vi "TEST - Copy with Options.vi"(8 "error in (no error)":errorcluster) -> (0 "error out":errorcluster, 2 "pass":bool)   [LabVIEW 2020]
uses:
  <userlib>/_OpenG.lib/error/error.llb/openg_error.lvlib
  source/library/openg_file.lvlib
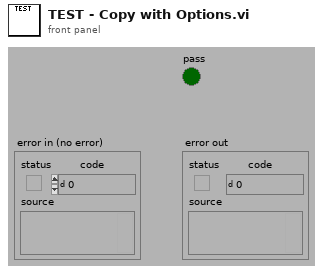
[diagram p1: front panel]
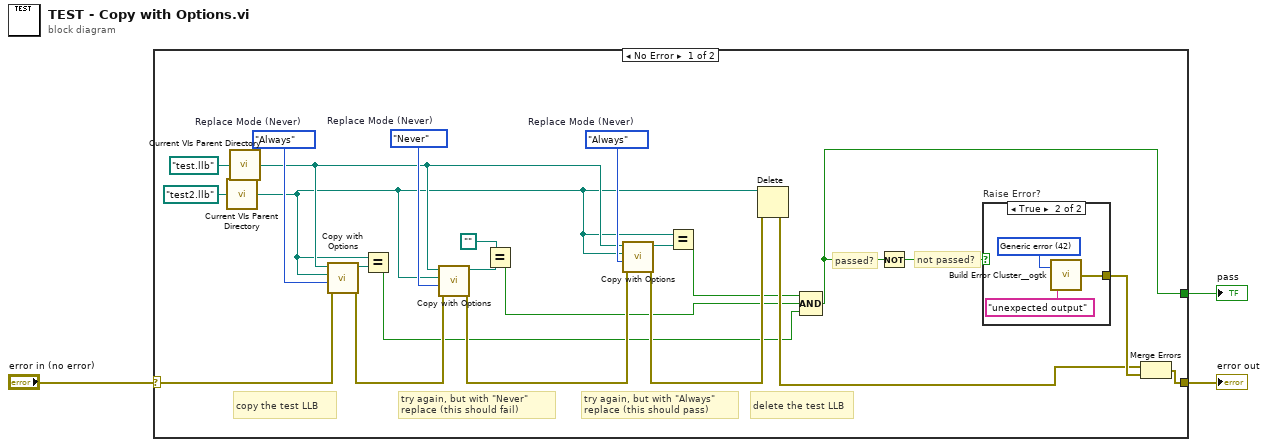
[diagram p0: block diagram]
diagram:
  n1 = case shown="No Error" "error in (no error)" {
    selector: "error in (no error)" -> [w22 w30]
    tunnel: [w18 _] -> w3
    tunnel: [w26 w30] -> w1
    frame No Error {
      w17 = enum16{"Never", "Always", "If Newer"}."Always"  # Replace Mode (Never)
      w19 = enum16{"Never", "Always", "If Newer"}."Always"  # Replace Mode (Never)
      w20 = enum16{"Never", "Always", "If Newer"}."Never"  # Replace Mode (Never)
      # "try again, but with \"Always\" replace (this should pass)"
      # "try again, but with \"Never\" replace (this should fail)"
      # "copy the test LLB"
      # "delete the test LLB"
      # "not passed?"
      # "passed?"
      n2 = call "Current VIs Parent Directory.vi"("Relative path (.)"=path "test2.llb") -> ("Parent Directory (+ Relative)"=w7:path)  [unwired: 4 in]
      n3 = call "Current VIs Parent Directory.vi"("Relative path (.)"=path "test.llb") -> ("Parent Directory (+ Relative)"=w14:path)  [unwired: 4 in]
      n4 = call "Copy with Options.vi"("error in (no error)"=w22, "Replace Mode (Never)"=w19, "target path"=w7, "source path"=w14) -> ("error out"=w21:errorcluster, "new path"=w9:path)  [unwired: 6 in]
      n5 = Equal?(x=w7, y=w9) -> (x = y?=w6:bool)
      n6 = call "Copy with Options.vi"("error in (no error)"=w21, "Replace Mode (Never)"=w20, "target path"=w7, "source path"=w14) -> ("error out"=w12:errorcluster, "new path"=w11:path)  [unwired: 6 in]
      n7 = Equal?(x=path "", y=w11) -> (x = y?=w5:bool)
      n8 = call "Copy with Options.vi"("error in (no error)"=w12, "Replace Mode (Never)"=w17, "target path"=w7, "source path"=w14) -> ("error out"=w16:errorcluster, "new path"=w8:path)  [unwired: 6 in]
      n9 = Equal?(x=w7, y=w8) -> (x = y?=w4:bool)
      n10 = Delete(path (use dialog)=w7, error in=w16) -> (error out=w23:errorcluster)  [unwired: 3 in, 2 out]
      n11 = Compound Arithmetic op=AND(w4, w5, w6) -> (w18:bool)
      n12 = Not(x=w18) -> (.not. x?=w24:bool)
      n13 = case "Raise Error?" shown="True" w24 {
        tunnel: [_ w27] -> w25
        frame False {
        }
        frame True {
          w28 = 42 items=["No error", "Argument error", "Memory is full", "Out of zone", "End of file", "File already open", "Generic file I/O error", "File not found", "File permission error", "Disk is full", "Duplicate path", "Too many files open", "System feature not enabled", "Resource file not found", "Cannot add resource", "Resource not found", "Image not found", "Image memory error", "Pen does not exist", "Config type invalid", "Config token not found", "Config parse error", "Config memory error", "Bad external code format", "Bad external code offset", "External code not present", "Null window", "Destroy window error", "Null menu", "Print aborted", "Bad print record", "Print driver error", "Windows error during printing", "Memory error during printing", "Print dialog error", "Generic print error", "Invalid device refnum", "Device not found", "Device parameter error", "Device unit error", "Cannot open device", "Device call aborted", "Generic error", "Cancelled by user", "Object ID too low", "Object ID too high", "Object not in heap", "Unknown heap", "Unknown object (invalid DefProc)", "Unknown object (DefProc not in table)", "Message out of range", "Invalid (null) method", "Unknown message", "Manager call not supported", "Bad address", "Network operation in progress", "Network operation timed out", "Connection is busy", "Network attribute not supported", "Network error", "Address in use", "System out of memory", "Connection aborted", "Connection refused", "Not connected", "Already connected", "Connection closed", "Initialization error (interapplication manager)", "Bad occurrence", "Wait on unbound occurrence handler", "Occurrence queue overflow", "Datalog type conflict", "Unused", "Unrecognized type (interapplication manager)", "Memory corrupt", "Failed to make temporary DLL", "Old CIN version", "Drag socket not found", "Failed to load drop-object", "Failed to register OLE object", "Failed to release OLE object", "Format specifier type mismatch", "Unknown format specifier", "Too few format specifiers", "Too many format specifiers", "Scan failed", "Newer CIN version", "Error converting to variant", "Runtime menu error", "Password tampered", "Variant attribute not found", "Incompatible variant data type", "Event data is not available", "Event Store is not present", "Occurrence is not found", "Event Queue is not created", "Event info is not available", "Refnum passed is NULL", "Error retrieving Class GUID", "Error retrieving CoClass GUID", "Error retrieving TypeLib GUID.", "Bad built application magic bytes.", "Specific driver is different from the specific driver associated with the Logical Name.", "There is no session opened to the class driver.", "Max Error", "MAX - Error with config objects", "MAX - Error loading configuration", "MAX - Group not supported"]
          n14 = call <userlib>:"Build Error Cluster__ogtk.vi"("String to Prepend to source (\"\")"="unexpected output" ("String to Prepend to source (\"\")"), "code"=w28) -> ("error out"=w27:errorcluster)
        }
      }
      n15 = Merge Errors(w23, w25) -> (w26:errorcluster)
    }
    frame Error {
    }
  }
  "pass" <- w3
  "error out" <- w1
